vi "连接断开动作.vi"(0 "MainPage 输入":refnum<class "MainPage.lvclass">) -> ()   [LabVIEW 2019, in "MainPage.lvlib" / "MainPage.lvclass"]
uses:
  MainPage.lvclass
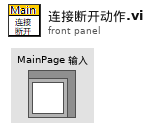
[diagram p1: front panel]
types:
  T1 = typedef "MainPage.lvlib/MainPage.lvclass/DataRef_通讯接口.ctl" = cluster{"连接方式":enum16{"网口(客服端)", "网口(服务端)", "串口"}, "VISA串口名称":refnum<visa-resource-name>, "服务端识别":cluster{"本机IP":string, "本机端口":u16, "当前目标":string}, "客服端识别":cluster{"客P-主IP:Port":string}, "服务端记录":cluster{"服务端侦听ID":refnum<k5>, "服务端接口记录":map{string, refnum<k5>}}, "客服端记录":map{string, refnum<k5>}}
  T2 = enum16{"ini", "增加记录", "读取记录", "更改寄存器值", "更改接口状态", "更改报文信息", "增加报文信息", "删除指定记录"}
  T3 = enum16{"ini", "读取", "写入-报文记录", "写入-寄存器模拟", "写入-串口状态", "增加报文记录"}
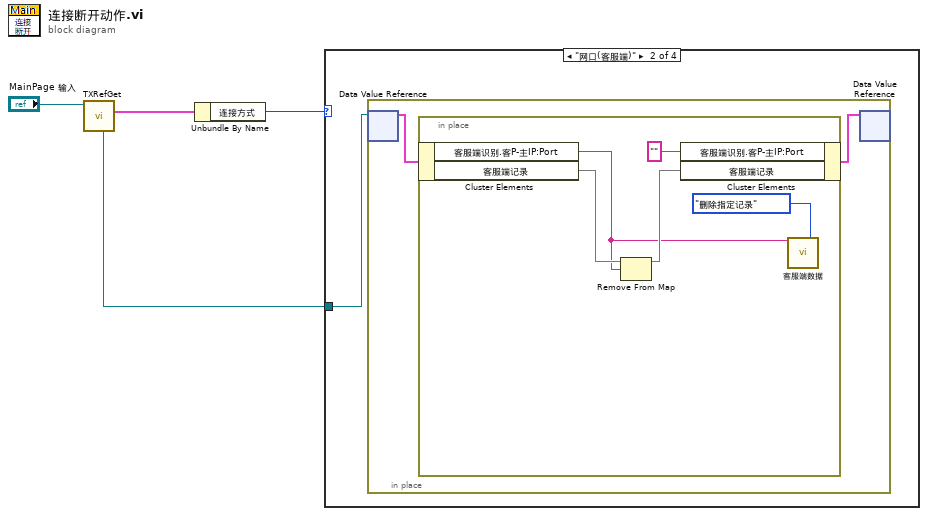
[diagram p0: block diagram]
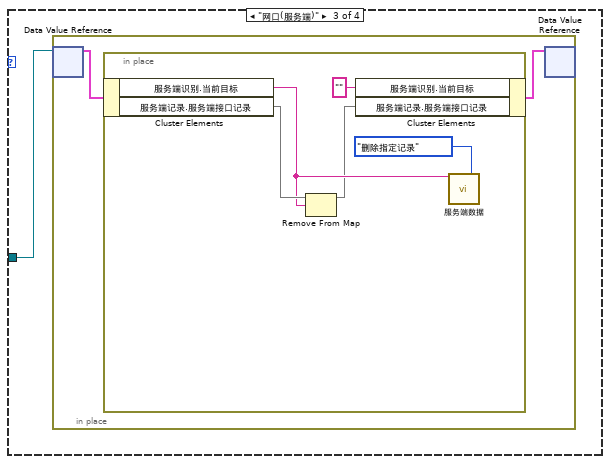
[diagram p3: hidden frame]
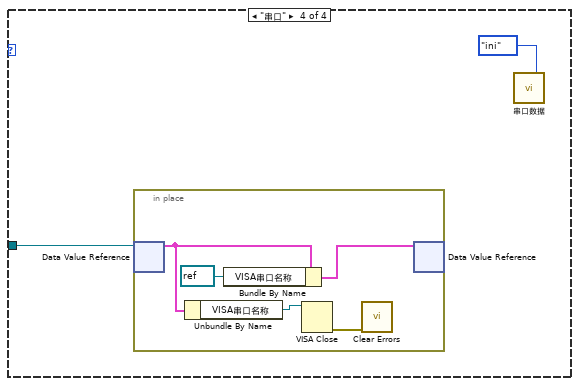
[diagram p4: hidden frame]
diagram:
  n1 = call-dynamic "TXRefGet.vi"("MainPage 输入"="MainPage 输入") -> ("通讯接口数据"=w3:T1, "引用"=w1:refnum<data-value>)  [unwired: 6 in, 3 out]
  n2 = Unbundle By Name(w3) -> ("连接方式"=w2:enum16{"网口(客服端)", "网口(服务端)", "串口"})
  n3 = case shown="\"网口(客服端)\"" w2 {
    tunnel: w1 -> [_ w5 w13 w21]
    frame Default {
    }
    frame "网口(客服端)" {
      n4 = in-place {
        n5 = in-place-dvr #1(w5) -> (w7:T1)  [unwired: 1 out]
        n6 = in-place {
          n7 = in-place-cluster #2(w7) -> ("客服端识别.客P-主IP:Port"=w8:string, "客服端记录"=w11:map{string, refnum<k5>})
          n8 = Remove From Map(10:w8, 11:w11) -> (3:w10:map{string, refnum<k5>})  [unwired: 2 out]
          n9 = in-place-cluster #2("客服端识别.客P-主IP:Port"="" ("服务端识别.当前目标"), "客服端记录"=w10) -> (w6:T1)
          n10 = call "客服端数据.vi"("客P-主IP:P"=w8, "枚举"=T2."删除指定记录") -> ()  [unwired: 16 in, 2 out]
        }
        n11 = in-place-dvr #1(w6) -> ()  [unwired: 2 out]
      }
    }
    frame "网口(服务端)" {
      n12 = in-place {
        n13 = in-place-dvr #3(w13) -> (w15:T1)  [unwired: 1 out]
        n14 = in-place {
          n15 = in-place-cluster #4(w15) -> ("服务端识别.当前目标"=w17:string, "服务端记录.服务端接口记录"=w18:map{string, refnum<k5>})
          n16 = Remove From Map(10:w17, 11:w18) -> (3:w16:map{string, refnum<k5>})  [unwired: 2 out]
          n17 = in-place-cluster #4("服务端识别.当前目标"="", "服务端记录.服务端接口记录"=w16) -> (w14:T1)
          n18 = call "服务端数据.vi"("IP-Port"=w17, "枚举"=T2."删除指定记录") -> ()  [unwired: 16 in, 2 out]
        }
        n19 = in-place-dvr #3(w14) -> ()  [unwired: 2 out]
      }
    }
    frame "串口" {
      n20 = in-place {
        n21 = in-place-dvr #5(w21) -> (w25:T1)  [unwired: 1 out]
        n22 = Unbundle By Name(w25) -> ("VISA串口名称"=w24:refnum<visa-resource-name>)
        n23 = Bundle By Name(cluster=w25, "VISA串口名称"=refnum<visa-resource-name> refnum) -> (w26:T1)
        n24 = VISA Close(VISA resource name=w24) -> (error out=w23:errorcluster)  [unwired: 1 in]
        n25 = call <vilib>:"Clear Errors.vi"("error in (no error)"=w23) -> ()  [unwired: 5 in, 2 out]
        n26 = in-place-dvr #5(w26) -> ()  [unwired: 2 out]
      }
      n27 = call "串口数据.vi"("枚举"=T3."ini") -> ()  [unwired: 18 in, 1 out]
    }
  }
